vi "Acquire.vi"(8 "error in (no error)":errorcluster, 9 "Data Queue":refnum<queue>, 10 "Data Notifier":refnum<notifier>, 11 "Hardware Resources in":T1={"AIDAQ"="", "Signal Type"=enum."Sine Wave", "DODAQ"=""}) -> (0 "error out":errorcluster, 3 "Hardware Resources out":T1={"AIDAQ"="", "Signal Type"=enum."Sine Wave", "DODAQ"=""})   [LabVIEW 2023, in "Acquisition.lvlib"]
doc: "Perform the acquisition. Replace the contents of this diagram with calls to acquisition hardware."
uses:
  Acquisition.lvlib
  Hardware Configuration.ctl
  Signal Type.ctl
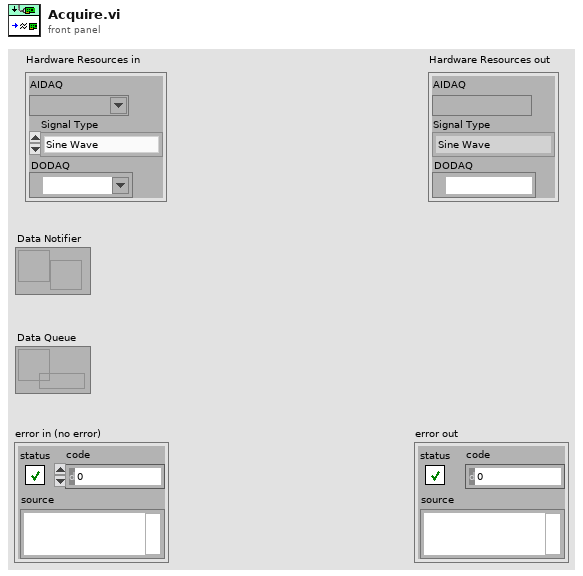
[diagram p1: front panel]
types:
  T1 = typedef "Acquisition.lvlib/Hardware Configuration.ctl" = cluster{"AIDAQ":refnum<k21>, "Signal Type":T2, "DODAQ":refnum<k21>}
  T2 = typedef "Acquisition.lvlib/Signal Type.ctl" = enum16{"cDAQ RTD", "myDAQ Temp", "Sine Wave", "Square with Noise"}
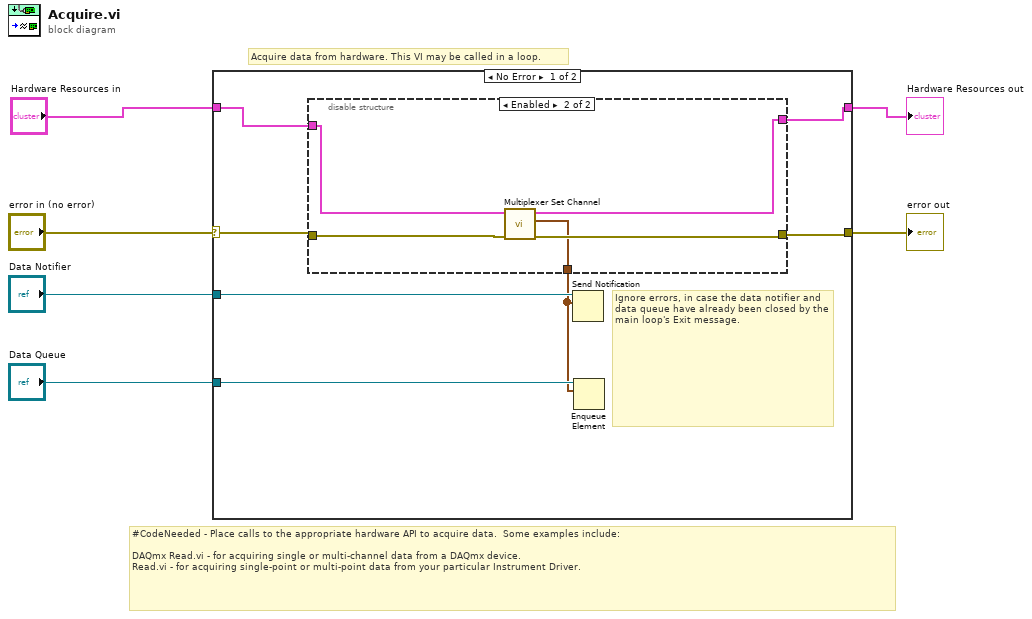
[diagram p0: block diagram]
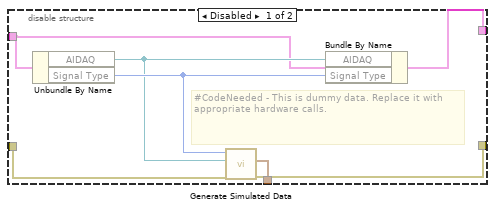
[diagram p2: hidden frame]
diagram:
  # "Acquire data from hardware. This VI may be called in a loop."
  # "#CodeNeeded - Place calls to the appropriate hardware API to acquire data.  Some examples include:\n\nDAQmx Read.vi - for acquiring single or multi-channel data from a DAQmx device.\nRead.vi - for acquiring single-point or multi-point data from your particular Instrument Driver."
  n1 = case shown="No Error" "error in (no error)" {
    selector: "error in (no error)" -> [w8 w26]
    tunnel: [w7 w26] -> w5
    tunnel: "Hardware Resources in" -> [w10 w27]
    tunnel: [w9 w27] -> w3
    tunnel: "Data Notifier" -> [w13 _]
    tunnel: "Data Queue" -> [w12 _]
    frame No Error {
      # "Ignore errors, in case the data notifier and data queue have already been closed by the main loop's Exit message."
      n2 = disable-structure shown="Enabled" {
        disable-tunnel: [w20 w22] -> w9
        disable-tunnel: [w18 w21] -> w11
        disable-tunnel: [w17 w24] -> w7
        disable-tunnel: w8 -> [w15 w25]
        disable-tunnel: w10 -> [w14 w23]
        frame Disabled {
          # "#CodeNeeded - This is dummy data. Replace it with appropriate hardware calls."
          n3 = Unbundle By Name(w14) -> ("AIDAQ"=w16:refnum<k21>, "Signal Type"=w19:T2)
          n4 = call "Generate Simulated Data.vi"("error in (no error)"=w15, "DAQmx Task Name"=w16, "Signal Type"=w19) -> ("error out"=w17:errorcluster, "Graph Data"=w18:waveform(dbl)[])  [unwired: 7 in]
          n5 = Bundle By Name(cluster=w14, "AIDAQ"=w16, "Signal Type"=w19) -> (w20:T1)
        }
        frame Enabled {
          n6 = call "Multiplexer Set Channel.vi"("error in (no error)"=w25, "Hardware Resources in"=w23) -> ("error out"=w24:errorcluster, "Graph Data"=w21:waveform(dbl)[], "Hardware Resources out"=w22:T1)  [unwired: 7 in]
        }
      }
      n7 = Send Notification(notification=w11, notifier=w13) -> ()  [unwired: 1 in, 2 out]
      n8 = Enqueue Element(queue=w12, element=w11) -> ()  [unwired: 2 in, 3 out]
    }
    frame Error {
    }
  }
  "Hardware Resources out" <- w3
  "error out" <- w5
